vi "TELOPS-DataFlow.vi"() -> ()   [LabVIEW 2011]
uses:
  <vilib>/Analysis/5stat.llb/RMS (DBL).vi
  <vilib>/Analysis/NI_AALBase.lvlib
  <vilib>/Analysis/NI_AALPro.lvlib
panel:
  in  "Only Servo ?":bool
  out "Eff. Ratio":dbl
  out "RMS COMMAND":dbl format="%.6f"
  out "RMS ERROR":dbl format="%.6f"
  out "XY Graph":T1(graph)
  out "Number of Lines":i32
  out "LineSize":i32
  out "Centroids":cluster{dbl[], dbl[]}[](graph)
  out "Flux":cluster{dbl[], dbl[]}[](graph)
  out "SNR":cluster{dbl[], dbl[]}[](graph)
  in  "Target ExecTime":u32=25
  in  "DataLenght":dbl
  out "HexpodXGraph":cluster{dbl[], dbl[]}[](graph)
  in  "DirPath":path=path "C:/BonOMM/BonOMM-2012/Syslogs/Hexapod/CommandLoggingClosedLoop"
  out "Cumulatif":cluster{dbl[], dbl[]}[](graph)
  out "ExecTime":u32=45
  out "HexapodYGraph":cluster{dbl[], dbl[]}[](graph)
  in  "Quit":bool
  # "FalconProcessed"
  # "CommandLogging"
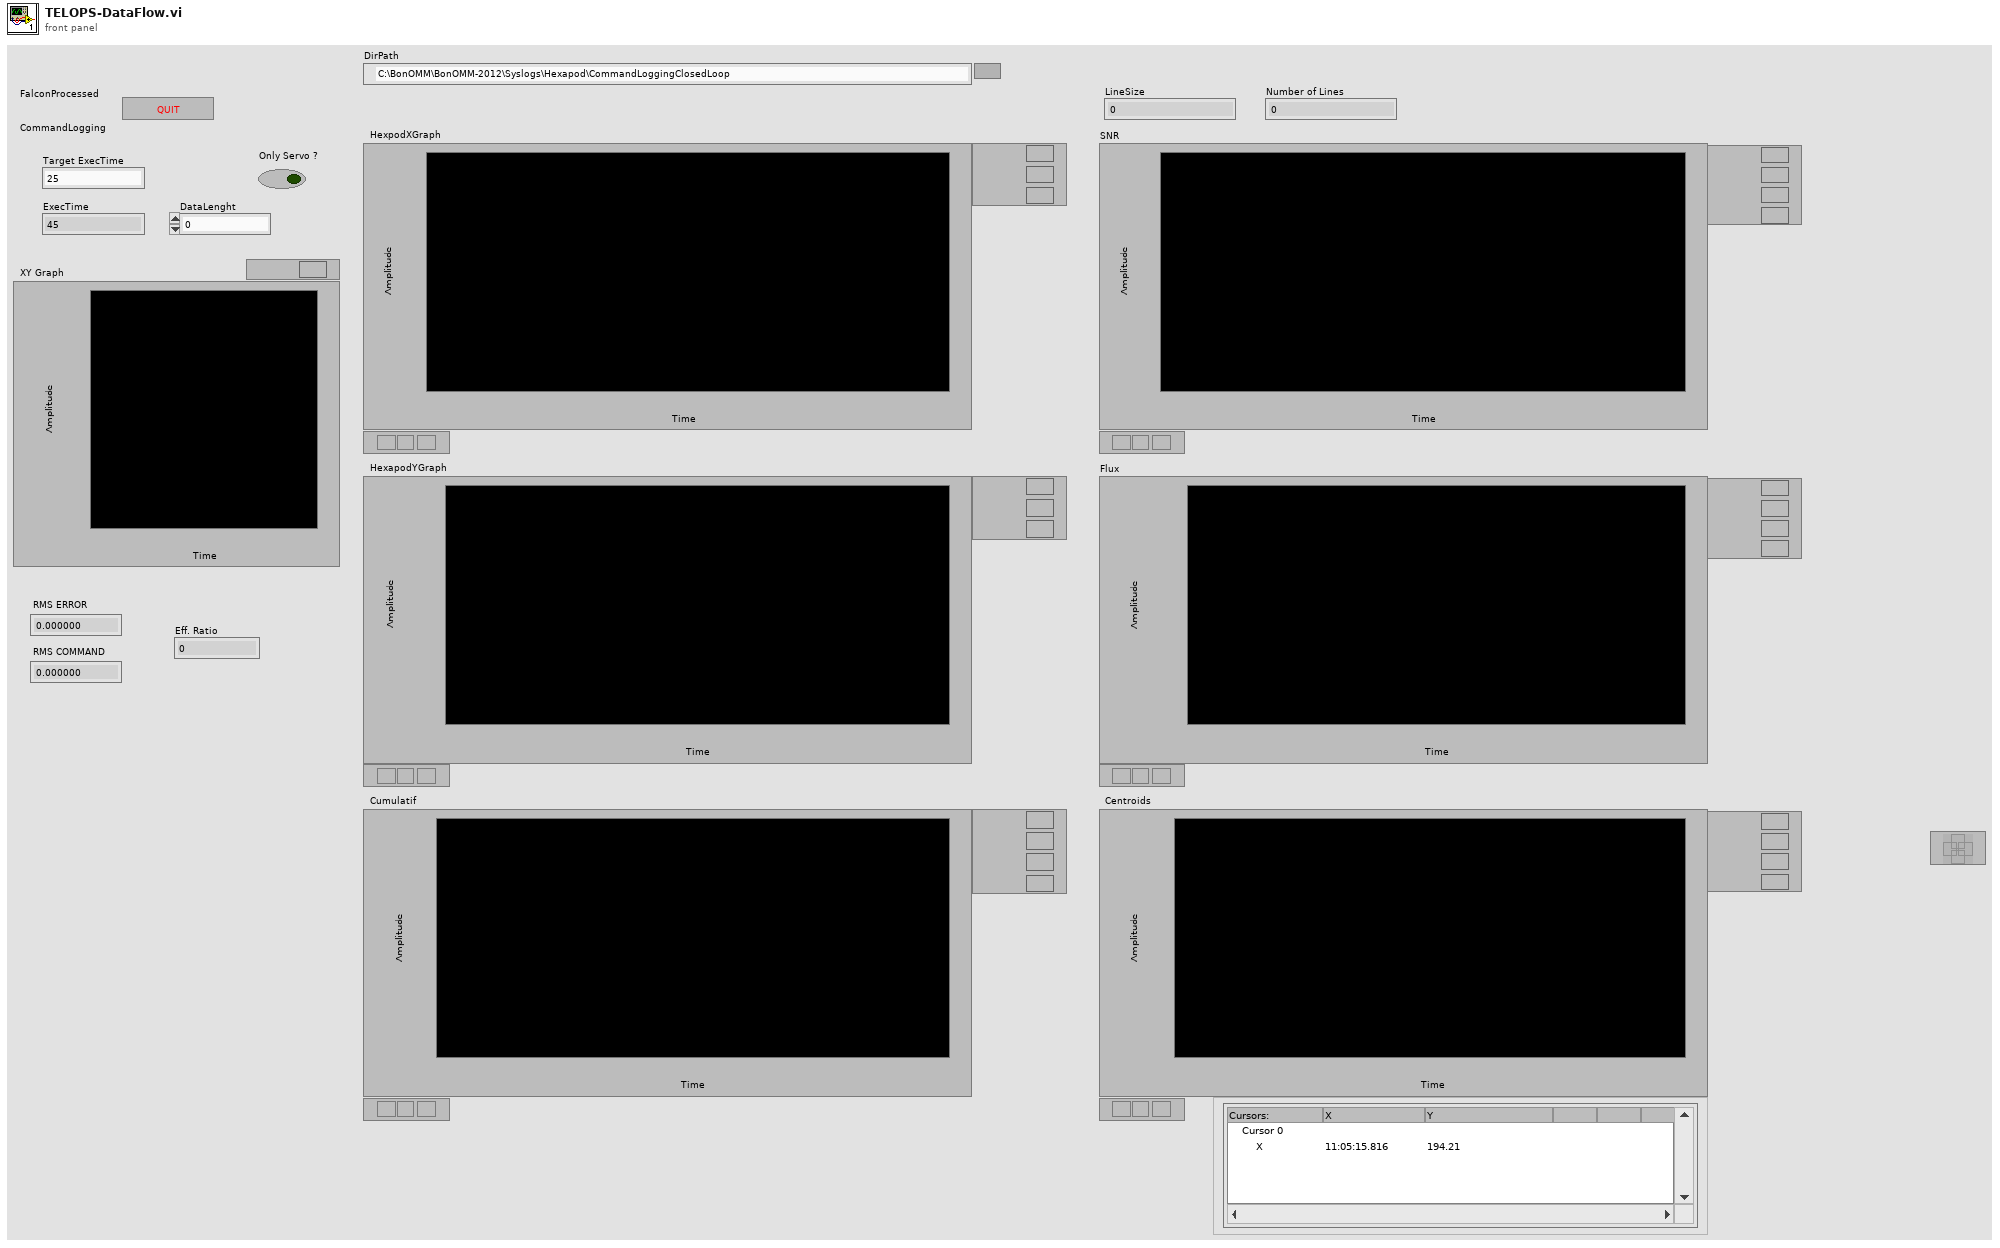
[diagram p1: front panel]
types:
  T1 = cluster{"X Values":dbl[], "Histogram: h(x)":i32[]}
  T2 = cluster{"Logging ID":u32, "Logging TimeStapmp":u64, "Azimuth":dbl, "Elevation":dbl, "Rotation":dbl, "ServoLevel":u16, "ROIWidth":u16, "ROIHeight":u16, "ROIXOffset":u16, "ROIYOffset":u16, "Pixel X":dbl, "Pixel Y":dbl, "ImageTimeStamp":u64, "CommandTimeStamp":u64, "Flux":dbl, "SNR":dbl, "SNRTreshold":dbl, "CentroidX":dbl, "CentroidY":dbl}
  T3 = cluster{"Hexapod_Nominal":dbl[], "Hexapod_Offset":dbl[], "Hexapod_LUT":dbl[], "Hexapod_ServoX":dbl[], "Hexapode_ServoY":dbl[], "Hexapod_Console":dbl[], "Hexapod_Position":dbl[], "Hexapod_Command":dbl[], "Hexapod_Filtered":dbl[]}
  T4 = cluster{"ROIXOffset":u16, "CentroidX":dbl, "Pixel X":dbl, "ROIYOffset":u16, "CentroidY":dbl, "Pixel Y":dbl}
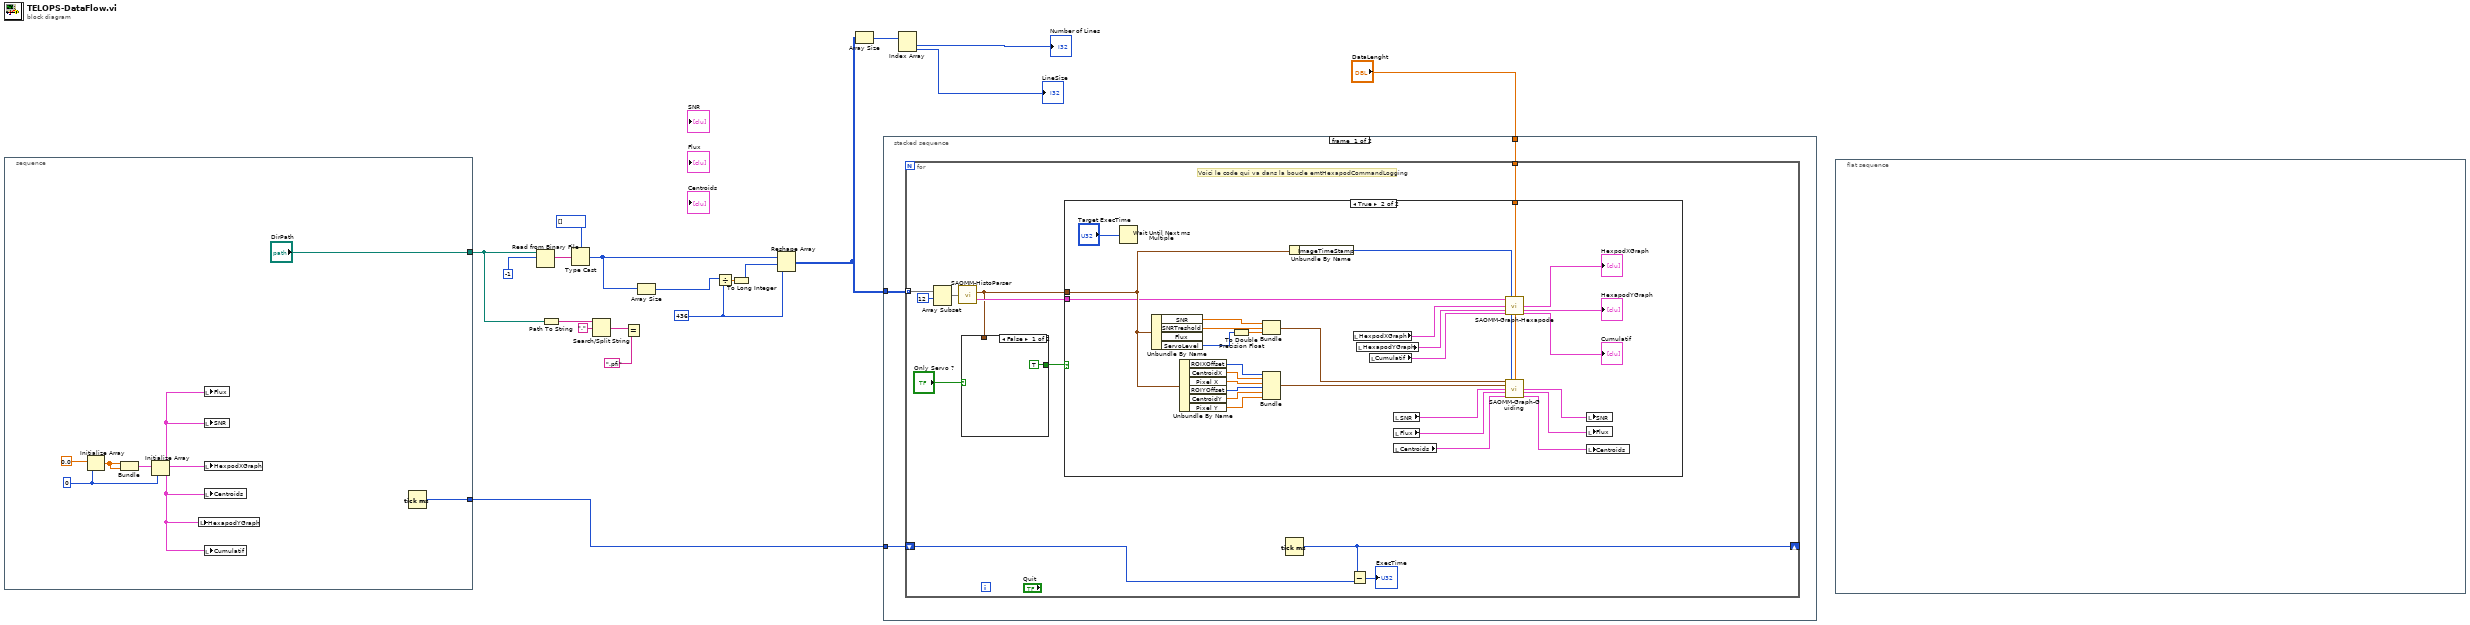
[diagram p0: block diagram]
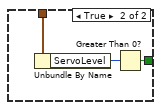
[diagram p3: hidden frame]
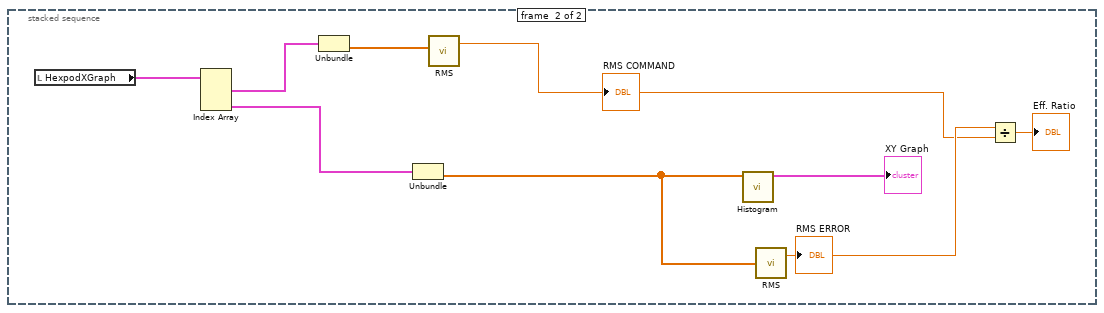
[diagram p4: hidden frame]
diagram:
  w6 = 436 ("dimension size")
  n1 = stacked-sequence {
    tunnel: [w26] -> w19
    tunnel: ["DirPath"] -> w13
    frame #0 {
      w22 = 0 ("millisecond multiple")
      n2 = Initialize Array(0.0, w22) -> (w24:dbl[])
      n3 = Bundle(w24, w24) -> (w23:cluster{dbl[], dbl[]})  [unwired: 1 in]
      n4 = Initialize Array(w23, w22) -> (w21:cluster{dbl[], dbl[]}[])
      n5 = local write "HexapodYGraph"(w21) -> ()
      n6 = local write "Flux"(w21) -> ()
      n7 = local write "SNR"(w21) -> ()
      n8 = local write "HexpodXGraph"(w21) -> ()
      n9 = local write "Centroids"(w21) -> ()
      n10 = local write "Cumulatif"(w21) -> ()
      n11 = Tick Count (ms)() -> (millisecond timer value=w26:u32)
    }
  }
  n12 = Read from Binary File(10:-1, 11:w13) -> (2:w11:string)  [unwired: 4 in, 3 out]
  n13 = Path To String(path=w13) -> (string=w17:string)
  n14 = Type Cast(type=u8[] [], x=w11) -> (*(type *) &x=w9:u8[])
  n15 = Search/Split String(string=w17, search string/char (-)=".") -> (match + rest of string=w16:string)  [unwired: 1 in, 2 out]
  n16 = Equal?(x=w16, y=".pfi") -> ()  [unwired: 1 out]
  n17 = Array Size(array=w9) -> (size(s)=w8:i32)
  n18 = Divide(x=w8, y=w6) -> (x/y=w7:dbl)
  n19 = To Long Integer(number=w7) -> (32bit integer=w5:i32)
  n20 = Reshape Array(w9, w5, w6) -> (w3:u8[][])
  n21 = Array Size(array=w3) -> (size(s)=w4:i32[])
  n22 = stacked-sequence {
    tunnel: w19 -> [w29 _]
    tunnel: "DataLenght" -> [w28 _]
    tunnel: w3 -> [w27 _]
    frame #0 {
      n23 = for {
        shift-right: [w39] -> _
        shift-left: w29 -> [w40]
        tunnel: w28 -> [w37]
        tunnel: w27 -> [w36] mode=indexing
        # "Voici le code qui va dans la boucle emtHexapodCommandLogging"
        n24 = Array Subset(array=w36, index=12) -> (w34:u8[])  [unwired: 1 in]
        n25 = call "SAOMM-HistoParser.vi"("DataStream"=w34) -> ("Source cluster"=w32:T2, "Hexapod cluster"=w33:T3)  [unwired: 13 in]
        n26 = case shown="False" "Only Servo ?" {
          tunnel: w32 -> [_ w73]
          tunnel: [TRUE w71] -> w31
          frame False {
          }
          frame True {
            n27 = Unbundle By Name(w73) -> ("ServoLevel"=w72:u16)
            n28 = Greater Than 0?(x=w72) -> (x > 0?=w71:bool)
          }
        }
        n29 = case shown="True" w31 {
          tunnel: w37 -> [_ w60]
          tunnel: w32 -> [_ w43]
          tunnel: w33 -> [_ w42]
          frame False {
          }
          frame True {
            n30 = Wait Until Next ms Multiple(millisecond multiple="Target ExecTime") -> ()  [unwired: 1 out]
            n31 = Unbundle By Name(w43) -> ("SNR"=w54:dbl, "SNRTreshold"=w55:dbl, "ServoLevel"=w45:u16)  [unwired: 1 out]
            n32 = Unbundle By Name(w43) -> ("ROIXOffset"=w52:u16, "CentroidX"=w51:dbl, "Pixel X"=w50:dbl, "ROIYOffset"=w49:u16, "CentroidY"=w48:dbl, "Pixel Y"=w47:dbl)
            n33 = To Double Precision Float(number=w45) -> (double precision float=w44:dbl)
            n34 = Bundle("SNR"=w54, "SNRTreshold"=w55, w44) -> (w53:cluster{"SNR":dbl, "SNRTreshold":dbl, dbl})  [unwired: 1 in]
            n35 = Bundle("ROIXOffset"=w52, "CentroidX"=w51, "Pixel X"=w50, "ROIYOffset"=w49, "CentroidY"=w48, "Pixel Y"=w47) -> (w46:T4)  [unwired: 1 in]
            n36 = Unbundle By Name(w43) -> ("ImageTimeStamp"=w56:u64)
            n37 = local read "HexpodXGraph"() -> (w68:cluster{dbl[], dbl[]}[])
            n38 = local read "HexapodYGraph"() -> (w69:cluster{dbl[], dbl[]}[])
            n39 = local read "Cumulatif"() -> (w65:cluster{dbl[], dbl[]}[])
            n40 = local read "SNR"() -> (w63:cluster{dbl[], dbl[]}[])
            n41 = local read "Flux"() -> (w62:cluster{dbl[], dbl[]}[])
            n42 = local read "Centroids"() -> (w61:cluster{dbl[], dbl[]}[])
            n43 = call "SAOMM-Graph-Hexapode.vi"("Hexapod cluster"=w42, "LoggingTimeStamp"=w56, "DataLenght (seconds)"=w60, "X IN"=w68, "Y IN"=w69, "Cumul IN"=w65) -> ("X OUT"=→"HexpodXGraph":cluster{dbl[], dbl[]}[], "Y OUT"=→"HexapodYGraph":cluster{dbl[], dbl[]}[], "Cumul OUT"=→"Cumulatif":cluster{dbl[], dbl[]}[])  [unwired: 7 in]
            n44 = call "SAOMM-Graph-Guiding.vi"("SNR Data"=w53, "TimeStamp"=w56, "DataLenght (seconds)"=w60, "Centroids Data"=w46, "SNR IN"=w63, "Flux IN"=w62, "Centroids IN"=w61) -> ("SNR OUT"=w59:cluster{dbl[], dbl[]}[], "Flux OUT"=w58:cluster{dbl[], dbl[]}[], "Centroids OUT"=w57:cluster{dbl[], dbl[]}[])  [unwired: 6 in]
            n45 = local write "SNR"(w59) -> ()
            n46 = local write "Flux"(w58) -> ()
            n47 = local write "Centroids"(w57) -> ()
          }
        }
        n48 = Tick Count (ms)() -> (millisecond timer value=w39:u32)
        n49 = Subtract(x=w39, y=w40) -> (x-y=→"ExecTime":u32)
      }
    }
    frame #1 {
      n50 = local read "HexpodXGraph"() -> (w80:cluster{dbl[], dbl[]}[])
      n51 = Index Array(array=w80) -> (element #1=w78:cluster{dbl[], dbl[]}, element #3=w79:cluster{dbl[], dbl[]})  [unwired: 3 in, 1 out]
      n52 = Unbundle(w78) -> (w77:dbl[])  [unwired: 1 out]
      n53 = Unbundle(w79) -> (w82:dbl[])  [unwired: 1 out]
      n54 = call-poly <vilib>:"RMS.vi"("X"=w77) -> ("rms value"=w75:dbl)  [unwired: 1 out]
      "RMS COMMAND" <- w75
      n55 = call <vilib>:"Histogram.vi"("X"=w82) -> ("Histogram Graph"=→"XY Graph":T1)  [unwired: 7 in, 3 out]
      n56 = call-poly <vilib>:"RMS.vi"("X"=w82) -> ("rms value"=w76:dbl)  [unwired: 1 out]
      "RMS ERROR" <- w76
      n57 = Divide(x=w76, y=w75) -> (x/y=→"Eff. Ratio":dbl)
    }
  }
  n58 = Index Array(array=w4) -> (element #1=→"Number of Lines":i32, element #2=→"LineSize":i32)  [unwired: 2 in]
  n59 = flat-sequence {
    frame #0 {
    }
  }
